vi "Get DQMH Scripting UI.vi"(8 "error in":errorcluster, 10 "DQMH Tools":T1, 11 "Project in":refnum<class "Project.lvclass">) -> (0 "error out":errorcluster, 1 "Implemented?":bool, 2 "DQMH UI Path":path)   [LabVIEW 2020, in "Panther Dashboard.lvlib" / "Project.lvclass"]
uses:
  Project.lvclass
  Panther Dashboard/DQMH Tools Menu--enum.ctl
  Read Main App Inst Ref.vi
  Panther Dashboard/Panther Dashboard.lvlib
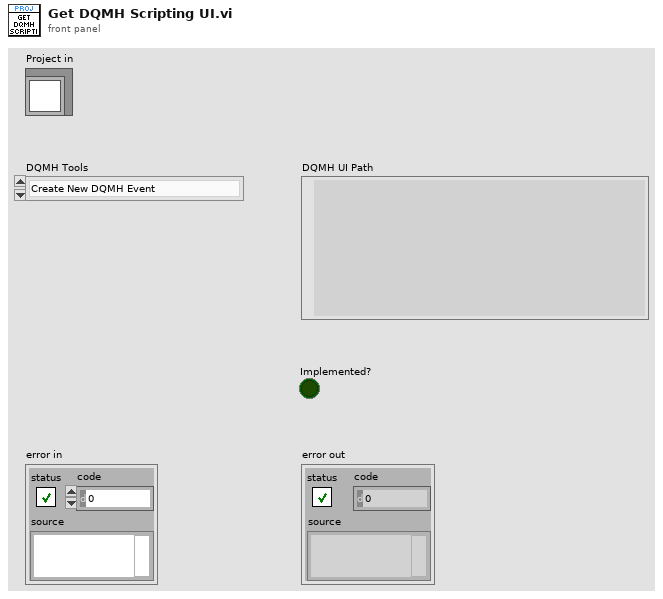
[diagram p1: front panel]
types:
  T1 = typedef "Panther Dashboard.lvlib/DQMH Tools Menu--enum.ctl" = enum16{"Create New DQMH Event", "Remove DQMH Event", "Convert DQMH Event", "Rename DQMH Event", "Add New DQMH Module", "Create RT Tester", "Rename DQMH Module", "Validate DQMH Module", "Create DQMH Module Template", "New DQMH  Unit Test", "Add Helper Loop to DQMH Module", "Duplicate Event", "HSE-ify DQMH Module", "Duplicate Module"}
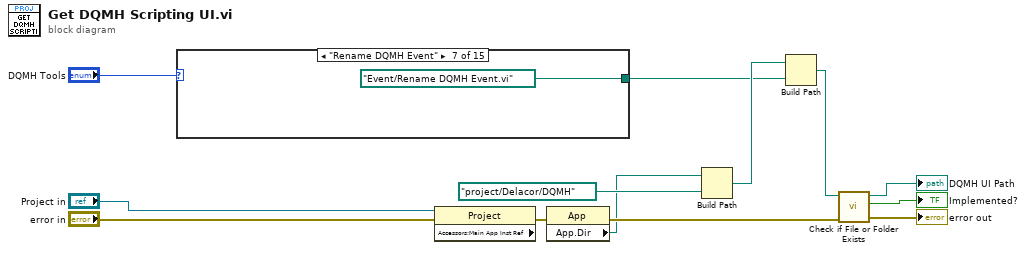
[diagram p0: block diagram]
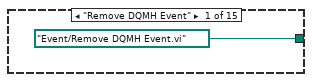
[diagram p2: hidden frame]
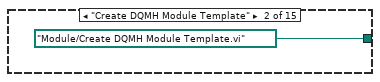
[diagram p3: hidden frame]
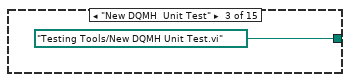
[diagram p4: hidden frame]
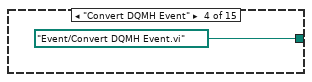
[diagram p5: hidden frame]
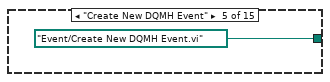
[diagram p6: hidden frame]
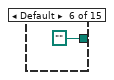
[diagram p7: hidden frame]
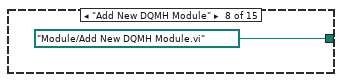
[diagram p8: hidden frame]
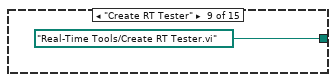
[diagram p9: hidden frame]
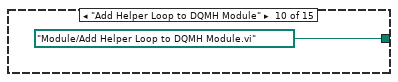
[diagram p10: hidden frame]
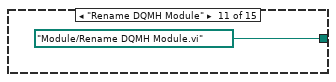
[diagram p11: hidden frame]
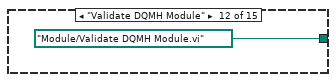
[diagram p12: hidden frame]
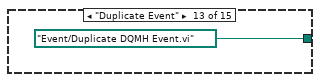
[diagram p13: hidden frame]
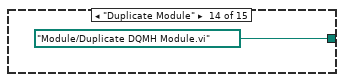
[diagram p14: hidden frame]
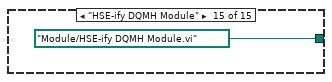
[diagram p15: hidden frame]
diagram:
  n1 = case shown="\"Rename DQMH Event\"" "DQMH Tools" {
    tunnel: [path "Event/Remove DQMH Event.vi" path "Module/Create DQMH Module Template.vi" path "Testing Tools/New DQMH Unit Test.vi" path "Event/Convert DQMH Event.vi" path "Event/Create New DQMH Event.vi" path "" path "Event/Rename DQMH Event.vi" path "Module/Add New DQMH Module.vi" path "Real-Time Tools/Create RT Tester.vi" path "Module/Add Helper Loop to DQMH Module.vi" path "Module/Rename DQMH Module.vi" path "Module/Validate DQMH Module.vi" path "Event/Duplicate DQMH Event.vi" path "Module/Duplicate DQMH Module.vi" path "Module/HSE-ify DQMH Module.vi"] -> w2
    frame "Remove DQMH Event" {
    }
    frame "Create DQMH Module Template" {
    }
    frame "New DQMH  Unit Test" {
    }
    frame "Convert DQMH Event" {
    }
    frame "Create New DQMH Event" {
    }
    frame Default {
    }
    frame "Rename DQMH Event" {
    }
    frame "Add New DQMH Module" {
    }
    frame "Create RT Tester" {
    }
    frame "Add Helper Loop to DQMH Module" {
    }
    frame "Rename DQMH Module" {
    }
    frame "Validate DQMH Module" {
    }
    frame "Duplicate Event" {
    }
    frame "Duplicate Module" {
    }
    frame "HSE-ify DQMH Module" {
    }
  }
  n2 = property class="Project" props=["Accessors:Main App Inst Ref"](reference="Project in", error in="error in") -> (error out=w12:errorcluster)  [unwired: 2 out]
  n3 = property class="App"(error in=w12) -> (error out=w11:errorcluster, "App.Dir"=w6:path)  [unwired: 1 in, 1 out]
  n4 = Build Path(base path=w6, name or relative path=path "project/Delacor/DQMH" ("Application:Directory Path")) -> (appended path=w7:path)
  n5 = Build Path(base path=w7, name or relative path=w2) -> (appended path=w1:path)
  n6 = call <vilib>:"Check if File or Folder Exists.vi"("error in (no error)"=w11, "path"=w1) -> ("error out"=→"error out":errorcluster, "file or folder exists?"=→"Implemented?":bool, "dup path"=→"DQMH UI Path":path)  [unwired: 7 in]
